vi "Provider_OnCommand.vi"(10 "Command ID":string, 11 "objects":T1[](array[typedef])) -> ()   [LabVIEW 2020, in "Actor Message Maker Provider.lvlib"]
uses:
  Actor Message Maker Provider.lvlib
  MessageMakerProvider/_Message Maker/Message Maker.lvlib
  <resource>/Framework/Providers/API/ItemRef.ctl
panel:
  out "error out":errorcluster
  in  "error in":errorcluster
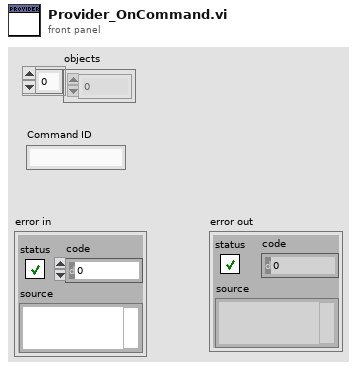
[diagram p1: front panel]
types:
  T1 = typedef "ItemRef.ctl" = u64
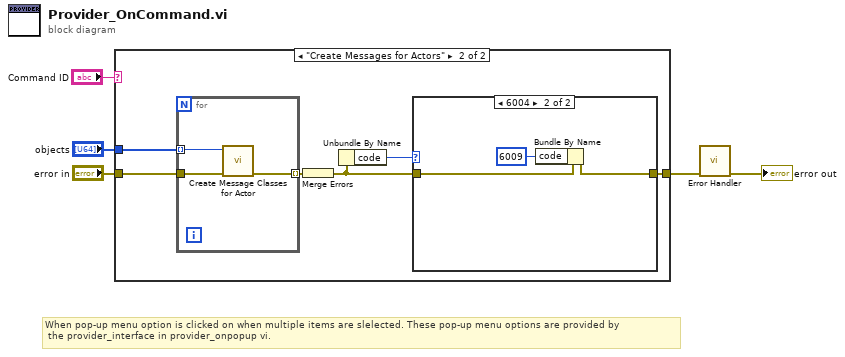
[diagram p0: block diagram]
diagram:
  # "When pop-up menu option is clicked on when multiple items are slelected. These pop-up menu options are provided by\n the provider_interface in provider_onpopup vi."
  n1 = case shown="\"Create Messages for Actors\"" "Command ID" {
    tunnel: "error in" -> [w6 w11]
    tunnel: [w6 w7] -> w2
    tunnel: "objects" -> [_ w12]
    frame Default {
    }
    frame "Create Messages for Actors" {
      n2 = for {
        tunnel: w12 -> [w19] mode=indexing
        tunnel: w11 -> [w18]
        tunnel: [w17] -> w10 mode=indexing
        n3 = call "Create Message Classes for Actor.vi"("error in (no error)"=w18, "Object"=w19) -> ("error out"=w17:errorcluster)  [unwired: 9 in]
      }
      n4 = Merge Errors(w10) -> (w8:errorcluster)
      n5 = Unbundle By Name(w8) -> ("code"=w9:i32)
      n6 = case shown="6004" w9 {
        tunnel: w8 -> [w13 w16]
        tunnel: [w13 w15] -> w7
        frame 0, Default {
        }
        frame 6004 {
          n7 = Bundle By Name(cluster=w16, "code"=6009) -> (w15:errorcluster)
        }
      }
    }
  }
  n8 = call "Error Handler.vi"("error in (no error)"=w2) -> ("error out"=→"error out":errorcluster)  [unwired: 10 in]
